vi "ANC300_communicate.vi"(0 "ANC300 Communication Port In":refnum<visa-resource-name>, 1 "connection ID in":refnum<k5>, 2 "commando string":string="ver()\n", 3 "Time to wait [ms]":u32=200, 4 "bytes to read":i32=200, 5 "error in":T1) -> (14 "ANC300 Communication Port Out":refnum<visa-resource-name>, 15 "connection ID out":refnum<k5>, 16 "read data":string, 17 "transfer ok":bool, 19 "error out":T1)   [LabVIEW 2023]
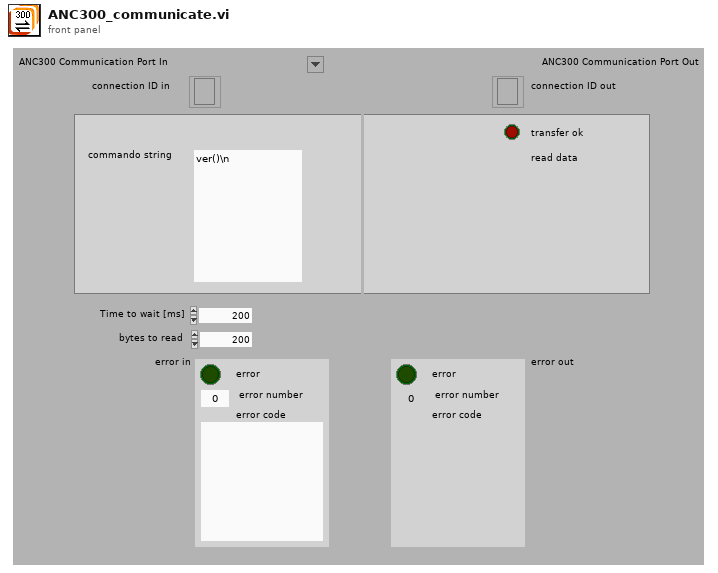
[diagram p1: front panel]
types:
  T1 = cluster{"error ":bool, "error number":i32, "error code":string}
  T2 = enum16{"Standard", "Buffered", "CRLF", "Immediate"}
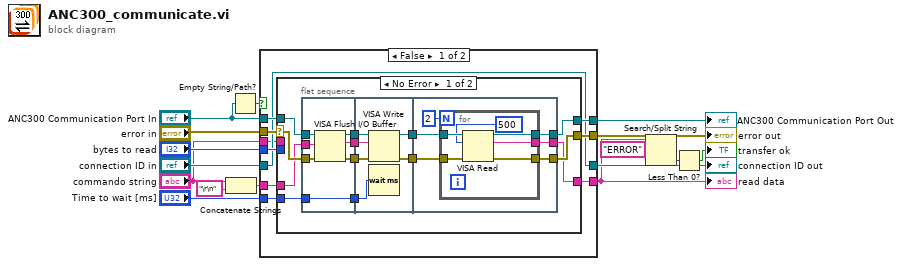
[diagram p0: block diagram]
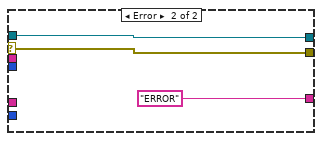
[diagram p2: hidden frame]
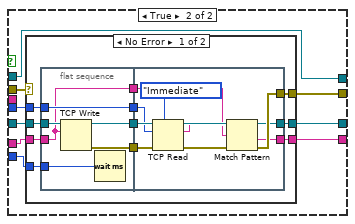
[diagram p3: hidden frame]
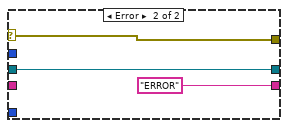
[diagram p4: hidden frame]
diagram:
  n1 = Concatenate Strings("commando string", "\r\n") -> (w3:string)
  n2 = Empty String/Path?(string/path="ANC300 Communication Port In") -> (empty?=w9:bool)
  n3 = case shown="False" w9 {
    tunnel: "connection ID in" -> [w18 w75]
    tunnel: w3 -> [w26 w74]
    tunnel: [w18 w73] -> w15
    tunnel: [w25 w72] -> w5
    tunnel: "bytes to read" -> [w24 w71]
    tunnel: "error in" -> [w23 w70]
    tunnel: [w22 w69] -> w12
    tunnel: "Time to wait [ms]" -> [w21 w67]
    tunnel: [w20 w68] -> w10
    tunnel: "ANC300 Communication Port In" -> [w19 w68]
    tunnel: "commando string" -> [w17 _]
    frame False {
      n4 = case shown="No Error" w23 {
        selector: w23 -> [w32 w66]
        tunnel: w26 -> [w31 _]
        tunnel: [w35 "ERROR"] -> w25
        tunnel: w24 -> [_ _]
        tunnel: [w36 w66] -> w22
        tunnel: w21 -> [w33 _]
        tunnel: [w37 w64] -> w20
        tunnel: w19 -> [w34 w64]
        tunnel: w17 -> [_ _]
        frame No Error {
          n5 = flat-sequence {
            tunnel: w33 -> [w44]
            tunnel: w31 -> [w45]
            tunnel: w32 -> [w40]
            tunnel: w34 -> [w43]
            tunnel: [w42] -> w30
            tunnel: [w41] -> w29
            tunnel: [w45] -> w28
            tunnel: [w44] -> w27
            tunnel: [w49] -> w39
            tunnel: [w48] -> w38
            tunnel: w30 -> [w51]
            tunnel: w29 -> [w50]
            tunnel: w28 -> [w46]
            tunnel: w27 -> [w47]
            tunnel: [w54] -> w35
            tunnel: [w55] -> w36
            tunnel: w39 -> [w57]
            tunnel: w38 -> [w56]
            tunnel: [w52] -> w37
            frame #0 {
              n6 = VISA Flush I/O Buffer(VISA resource name=w43, error in (no error)=w40) -> (VISA resource name out=w42:refnum<visa-resource-name>, error out=w41:errorcluster)  [unwired: 1 in]
            }
            frame #1 {
              n7 = VISA Write(VISA resource name=w51, write buffer=w46, error in (no error)=w50) -> (VISA resource name out=w49:refnum<visa-resource-name>, error out=w48:errorcluster)  [unwired: 1 out]
              n8 = Wait (ms)(milliseconds to wait=w47) -> ()  [unwired: 1 out]
            }
            frame #2 {
              n9 = for {
                N: 2 -> [_]
                tunnel: w57 -> [w63]
                tunnel: w56 -> [w62]
                tunnel: [w61] -> w55
                tunnel: [w60] -> w52
                tunnel: [w58] -> w54
                n10 = VISA Read(VISA resource name=w63, byte count=500, error in (no error)=w62) -> (VISA resource name out=w60:refnum<visa-resource-name>, read buffer=w58:string, error out=w61:errorcluster)  [unwired: 1 out]
              }
            }
          }
        }
        frame Error {
        }
      }
    }
    frame True {
      n11 = case shown="No Error" w70 {
        selector: w70 -> [_ w104]
        tunnel: w75 -> [w84 w103]
        tunnel: w74 -> [w83 _]
        tunnel: [w78 w103] -> w73
        tunnel: [w82 "ERROR"] -> w72
        tunnel: w71 -> [w81 _]
        tunnel: [w79 w104] -> w69
        tunnel: w67 -> [w76 _]
        frame No Error {
          n12 = flat-sequence {
            tunnel: [w92] -> w86
            tunnel: w84 -> [w91]
            tunnel: w83 -> [w88]
            tunnel: w81 -> [w90]
            tunnel: [w90] -> w85
            tunnel: [w89] -> w80
            tunnel: [w88] -> w77
            tunnel: w76 -> [w87]
            tunnel: [w93] -> w82
            tunnel: w86 -> [w101]
            tunnel: w85 -> [w99]
            tunnel: w80 -> [w100]
            tunnel: [w97] -> w79
            tunnel: [w96] -> w78
            tunnel: w77 -> [w94]
            frame #0 {
              n13 = TCP Write(connection ID=w91, data in=w88) -> (connection ID out=w92:refnum<k5>, error out=w89:errorcluster)  [unwired: 2 in, 1 out]
              n14 = Wait (ms)(milliseconds to wait=w87) -> ()  [unwired: 1 out]
            }
            frame #1 {
              n15 = TCP Read(connection ID=w101, bytes to read=w99, error in (no error)=w100, 7:T2."Immediate" ("mode (standard)")) -> (connection ID out=w96:refnum<k5>, data out=w95:string, error out=w97:errorcluster)  [unwired: 1 in]
              n16 = Match Pattern(string=w95, regular expression=w94) -> (after substring=w93:string)  [unwired: 1 in, 3 out]
            }
          }
        }
        frame Error {
        }
      }
    }
  }
  "connection ID out" <- w15
  "read data" <- w5
  "error out" <- w12
  "ANC300 Communication Port Out" <- w10
  n17 = Search/Split String(string=w5, search string/char (-)="ERROR") -> (offset of match=w7:i32)  [unwired: 1 in, 2 out]
  n18 = Less Than 0?(x=w7) -> (x < 0?=→"transfer ok":bool)
